vi "Output_Scaling.vi"(8 "Right Motor Voltage":dbl, 9 "Left Motor Voltage":dbl) -> (2 "Right Motor PWM (ticks)":i16, 3 "Left Motor PWM (ticks)":i16)   [LabVIEW 2019]
panel:
  in  "PWM Period (ticks)":i16=2000
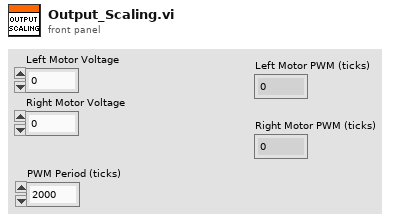
[diagram p1: front panel]
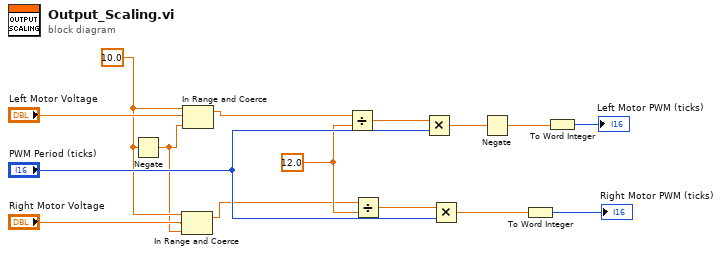
[diagram p0: block diagram]
diagram:
  w3 = 10.0
  w13 = 12.0 ("y")
  n1 = Negate(x=w3) -> (-x=w2:dbl)
  n2 = In Range and Coerce(upper limit=w3, x="Right Motor Voltage", lower limit=w2) -> (coerced(x)=w1:dbl)  [unwired: 1 out]
  n3 = In Range and Coerce(upper limit=w3, x="Left Motor Voltage", lower limit=w2) -> (coerced(x)=w6:dbl)  [unwired: 1 out]
  n4 = Divide(x=w6, y=w13) -> (x/y=w14:dbl)
  n5 = Divide(x=w1, y=w13) -> (x/y=w12:dbl)
  n6 = Multiply(x=w14, y="PWM Period (ticks)") -> (x*y=w10:dbl)
  n7 = Multiply ("Multiply 3")(x=w12, y="PWM Period (ticks)") -> (x*y=w9:dbl)
  n8 = Negate(x=w10) -> (-x=w11:dbl)
  n9 = To Word Integer ("To Word Integer 2")(number=w9) -> (16bit integer=→"Right Motor PWM (ticks)":i16)
  n10 = To Word Integer(number=w11) -> (16bit integer=→"Left Motor PWM (ticks)":i16)
